vi "tsc--Cancel Topmost.vi"(8 "Error In":errorcluster, 11 "This VI":refnum<vi>) -> (0 "Error Out":errorcluster)   [LabVIEW 2021]
doc: "Adapted from: https://lavag.org/topic/12751-how-do-you-make-your-application-window-frontmost/?do=findComment&comment=113072\n\nSets the Caller VIs front panel NoTopmost (above all non-topmost windows), thereby cancelling the TopMost setting.\n\nCopyright © 2010 Blue Ridge Test, Inc.\nwww.BlueRidgeTest.com"
uses:
  user32.dll
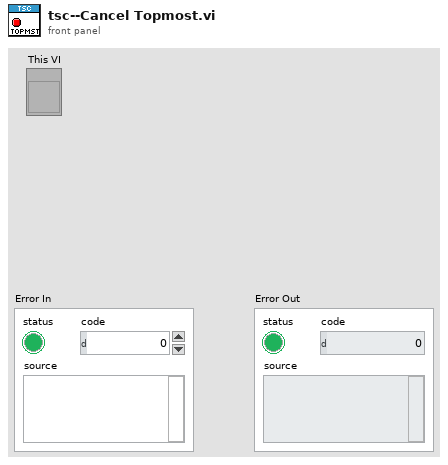
[diagram p1: front panel]
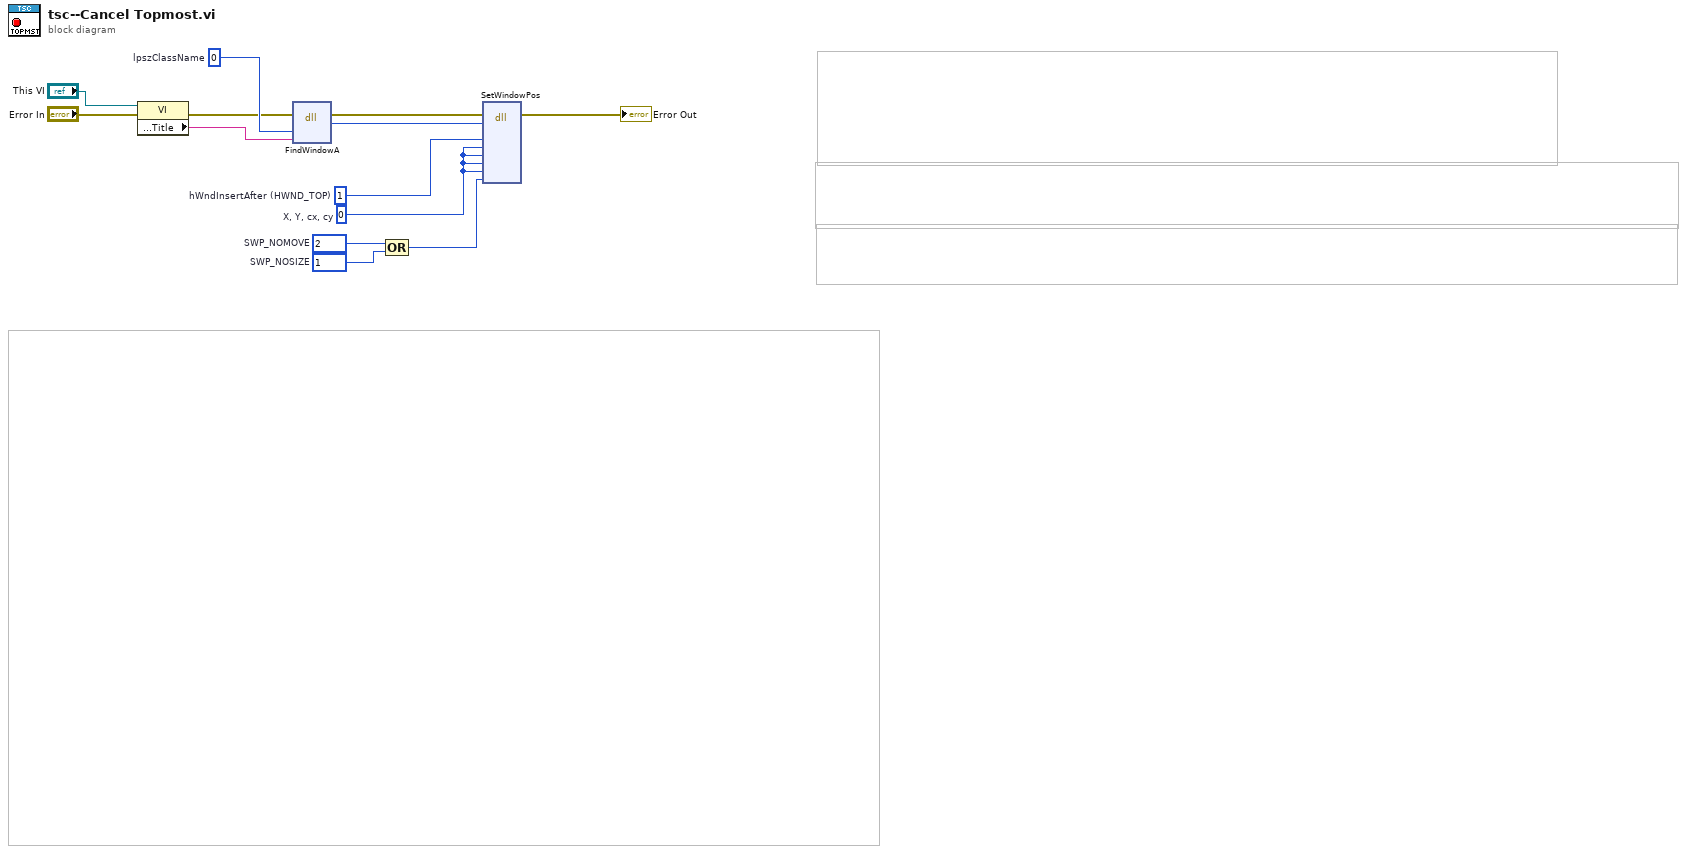
[diagram p0: block diagram]
diagram:
  w8 = 0  # lpszClassName
  w12 = 1  # hWndInsertAfter (HWND_TOP)
  w10 = u32 2  # SWP_NOMOVE
  w11 = u32 1  # SWP_NOSIZE
  w5 = 0  # X, Y, cx, cy
  n1 = property class="VI"(reference="This VI", error in="Error In") -> (error out=w3:errorcluster, "Front Panel.Title"=w2:string)  [unwired: 1 out]
  n2 = dll-call lib="user32.dll" fn="FindWindowA" label="FindWindow"(error in=w3, "lpszClassName"=w8, "lpszWindowName"=w2) -> (error out=w4:errorcluster, "hWnd"=w7:u32)  [unwired: 4 in, 1 out]
  n3 = Compound Arithmetic op=OR(w10, w11) -> (w6:u32)
  n4 = dll-call lib="USER32.DLL" fn="SetWindowPos"(error in=w4, "hWnd"=w7, "hWndInsertAfter"=w12, "left"=w5, "top"=w5, "width"=w5, "height"=w5, "fuFlags"=w6) -> (error out=→"Error Out":errorcluster)  [unwired: 8 in, 3 out]
